vi "Set Command Timeout.vi"(4 "error in":errorcluster, 6 "CommandTimeout":i32=30, 7 "Connection In":refnum<k7>) -> (0 "error out":errorcluster, 3 "Connection Out":refnum<k7>)   [LabVIEW 2022 SP3, in "hse-db-ado.lvlib" / "ADO-DB-Driver.lvlib"]
doc: "Set the command timeout\n\n____\nHAMPEL SOFTWARE ENGINEERING v1.4.0 (2023-12-19 09:52)"
uses:
  ADO-DB-Driver.lvlib
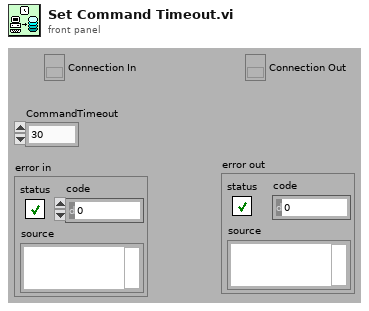
[diagram p1: front panel]
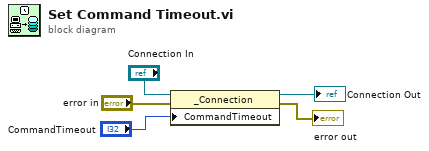
[diagram p0: block diagram]
diagram:
  n1 = property class="_Connection"(reference="Connection In", error in="error in", "CommandTimeout"="CommandTimeout") -> (reference out=→"Connection Out":refnum<k7>, error out=→"error out":errorcluster)
